vi "Clear_Info.vi"(8 "error in (no error)":errorcluster, 9 "index in":string, 10 "buildObject":T1, 11 "IB_Source_Container in":refnum<class "IB_Source_Container.lvclass">) -> (0 "error out":errorcluster, 1 "index out":string, 2 "buildObject out":T1, 3 "IB_Source_Container out":refnum<class "IB_Source_Container.lvclass">)   [LabVIEW 2020, in "IB_Source_Container.lvclass"]
uses:
  <vilib>/AppBuilder/IB_Classes/Source/Container/IB_Source_Container.lvclass
  <vilib>/AppBuilder/IB_Classes/Source/Container/IB_Source_Container.lvclass/IB_Source_Container.ctl
  <vilib>/AppBuilder/IB_Classes/Source/IB_Source.lvclass
  <vilib>/AppBuilder/IB_Classes/Source/File/CtrFile/IB_CtrFile.lvclass
  <resource>/Framework/Providers/API/ItemRef.ctl
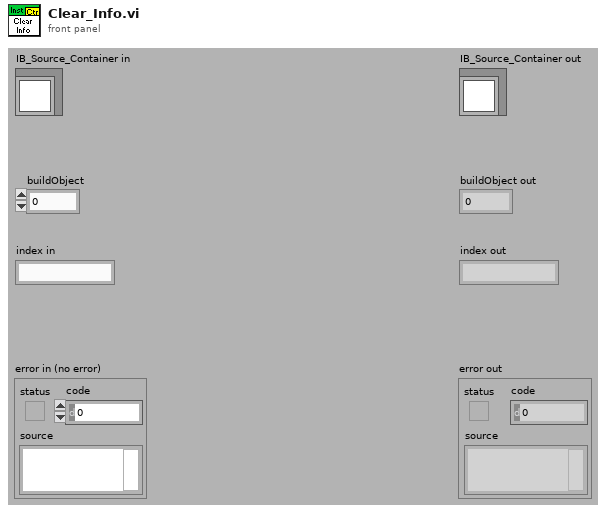
[diagram p1: front panel]
types:
  T1 = typedef "ItemRef.ctl" = u64
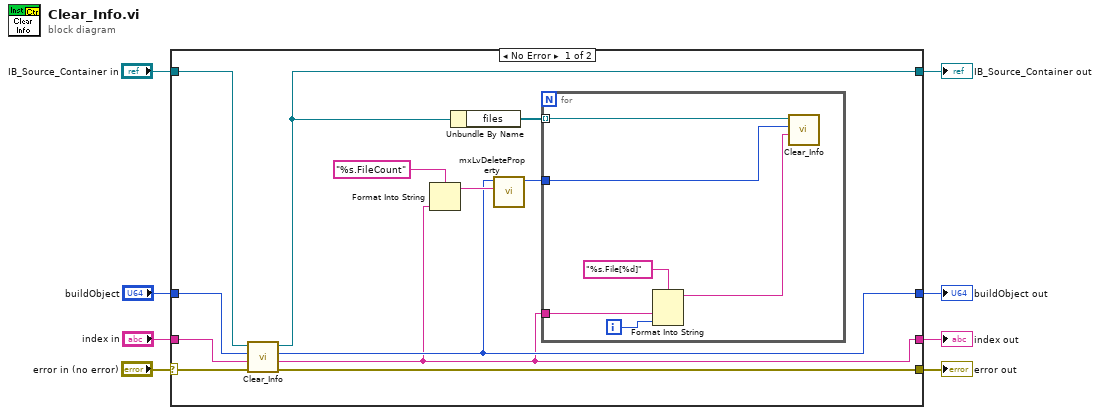
[diagram p0: block diagram]
diagram:
  n1 = case shown="No Error" "error in (no error)" {
    selector: "error in (no error)" -> [w16 w30]
    tunnel: [w20 w30] -> w8
    tunnel: [w9 w29] -> w7
    tunnel: [w12 w28] -> w6
    tunnel: [w10 w27] -> w5
    tunnel: "index in" -> [w19 w29]
    tunnel: "buildObject" -> [w18 w28]
    tunnel: "IB_Source_Container in" -> [w17 w27]
    frame No Error {
      n2 = call-parent "Clear_Info.vi"("error in (no error)"=w16, "index in"=w19, "buildObject"=w18, "IB_Source in"=w17) -> ("error out"=w20:errorcluster, "index out"=w9:string, "buildObject out"=w12:T1, "IB_Source out"=w10:refnum<class "IB_Source_Container.lvclass">)  [unwired: 4 in]
      n3 = Format Into String(format string="%s.FileCount", w9) -> (resulting string=w14:string)  [unwired: 2 in, 1 out]
      n4 = Unbundle By Name(w10) -> ("files"=w15:refnum<class "IB_CtrFile.lvclass">[])
      n5 = call <resource>:"mxLvDeleteProperty.vi"("Tag"=w14, "Item"=w12) -> ("Item"=w11:T1)  [unwired: 1 in, 8 out]
      n6 = for {
        tunnel: w15 -> [w26] mode=indexing
        tunnel: w11 -> [w25]
        tunnel: w9 -> [w23]
        i -> [w22]
        n7 = Format Into String(format string="%s.File[%d]", w23, w22) -> (resulting string=w21:string)  [unwired: 2 in, 1 out]
        n8 = call-dynamic "Clear_Info.vi"("index in"=w21, "buildObject"=w25, "IB_Source_File in"=w26) -> ()  [unwired: 5 in, 4 out]
      }
    }
    frame Error {
    }
  }
  "error out" <- w8
  "IB_Source_Container out" <- w5
  "buildObject out" <- w6
  "index out" <- w7
